vi "1 byte transfer.vi"(0 "Min time SCL low (uSec)":u32, 1 "Min Time SCL high (uSec)":u32, 2 "Data bit array":bool[](array[boolean])=[FALSE, FALSE, FALSE, FALSE, FALSE, FALSE, FALSE, FALSE]) -> ()   [LabVIEW 2019]
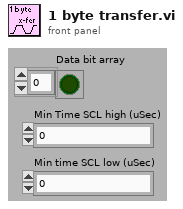
[diagram p1: front panel]
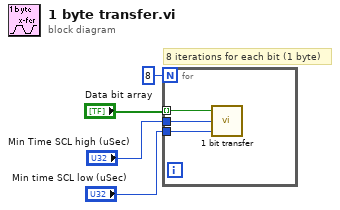
[diagram p0: block diagram]
diagram:
  # "8 iterations for each bit (1 byte)"
  n1 = for {
    N: 8 -> [_]
    tunnel: "Data bit array" -> [w7] mode=indexing
    tunnel: "Min Time SCL high (uSec)" -> [w6]
    tunnel: "Min time SCL low (uSec)" -> [w5]
    n2 = call "1 bit transfer.vi"("Min time SCL low (uSec)"=w5, "Min Time SCL high (uSec)"=w6, "Data bit"=w7) -> ()
  }
